vi "File_Build Save File Path.vi"(3 "File Name":string, 4 "File Keeper Files":T1=enum."PNG Image Folder") -> (5 "File Path Out":path)   [LabVIEW 2015]
uses:
  TypeDefs_Utility/ENUM_File Keeper List.ctl
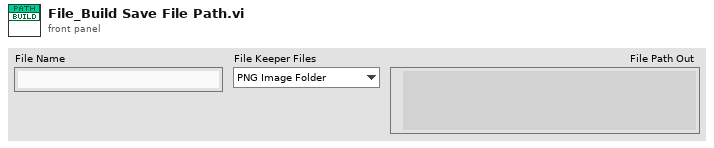
[diagram p1: front panel]
types:
  T1 = typedef "ENUM_File Keeper List.ctl" = enum16{"Calibration File Folder", "PNG Image Folder", "CSV File Folder"}
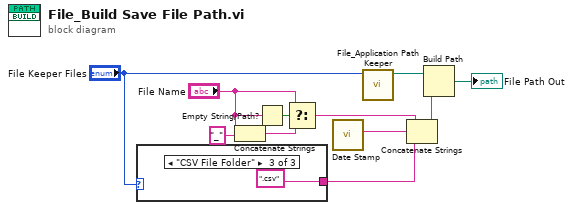
[diagram p0: block diagram]
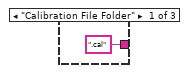
[diagram p2: hidden frame]
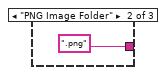
[diagram p3: hidden frame]
diagram:
  n1 = case shown="\"CSV File Folder\"" "File Keeper Files" {
    tunnel: [".cal" ("string") ".png" ("string") ".csv" ("string")] -> w11
    frame "Calibration File Folder" {
    }
    frame "PNG Image Folder" {
    }
    frame "CSV File Folder" {
    }
  }
  n2 = Concatenate Strings("File Name", "_" ("string")) -> (w2:string)
  n3 = Empty String/Path?(string/path="File Name") -> (empty?=w5:bool)
  n4 = Select(t="File Name", s=w5, f=w2) -> (s? t:f=w1:string)
  n5 = call "Date Stamp.vi"() -> ("String Out"=w9:string)  [unwired: 5 in, 1 out]
  n6 = call "File_Application Path Keeper.vi"("File Keeper Files"="File Keeper Files") -> ("Path Out"=w7:path)  [unwired: 8 in, 2 out]
  n7 = Concatenate Strings(w1, w9, w11) -> (w10:string)
  n8 = Build Path(base path=w7, name or relative path=w10) -> (appended path=→"File Path Out":path)
